vi "Coerce Steering Frame Velocity.vi"(8 "error in (no error)":errorcluster, 10 "steering frame velocity":dbl[](array[numeric])=[0.0, 0.0, 0.0], 11 "differential steering frame in":refnum<class "NI_Robotics_Differential Steering Frame.lvclass">) -> (0 "error out":errorcluster, 2 "coerced steering frame velocity":dbl[](array[numeric]), 3 "differential steering frame out":refnum<class "NI_Robotics_Differential Steering Frame.lvclass">)   [LabVIEW 2017, in "NI_Robotics_Differential Steering Frame.lvclass"]
doc: "Coerces the steering frame velocity to meet the constraints of the steering frame type. This VI does not coerce the velocity based on the constraints of individual wheels."
uses:
  <vilib>/robotics/Steering/Differential Steering Frame/NI_Robotics_Differential Steering Frame.lvclass
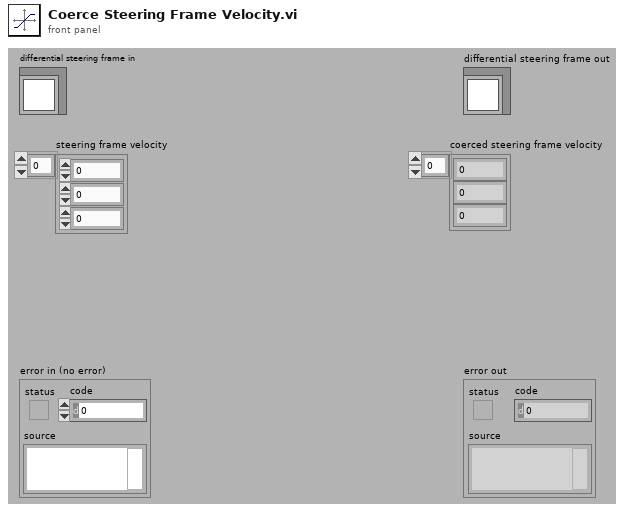
[diagram p1: front panel]
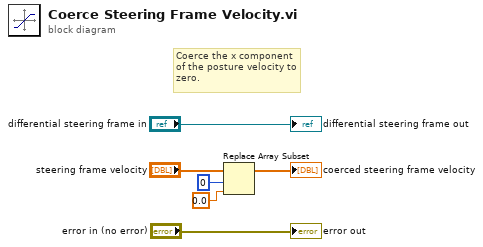
[diagram p0: block diagram]
diagram:
  # "Coerce the x component of the posture velocity to zero."
  n1 = Replace Array Subset(array="steering frame velocity", new element=0.0 ("new element/subarray"), index=0) -> (→"coerced steering frame velocity":dbl[])
  "error out" <- "error in (no error)"
  "differential steering frame out" <- "differential steering frame in"
